vi "Set Extension.vi"(8 "error in (no error)":errorcluster, 11 "Report in":refnum<class "Wind Report.lvclass">) -> (0 "error out":errorcluster, 3 "Report out":refnum<class "Wind Report.lvclass">)   [LabVIEW 2009, in "Wind Report.lvclass"]
doc: "The protected method in the Wind Report class sets the file extension type in the object data for child classes.\n\nAAL 9/09"
uses:
  Wind Report.lvclass
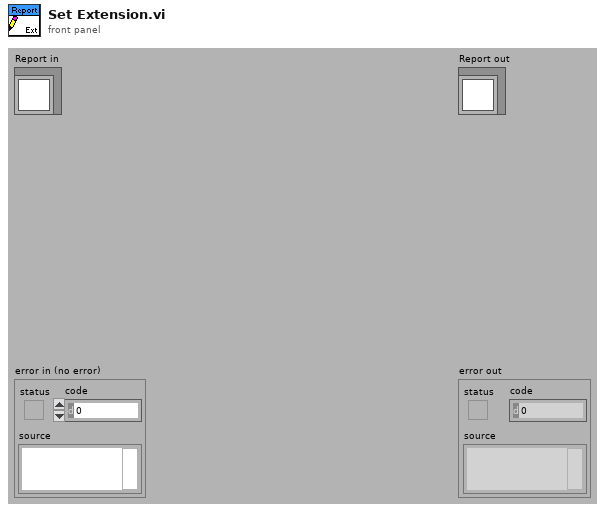
[diagram p1: front panel]
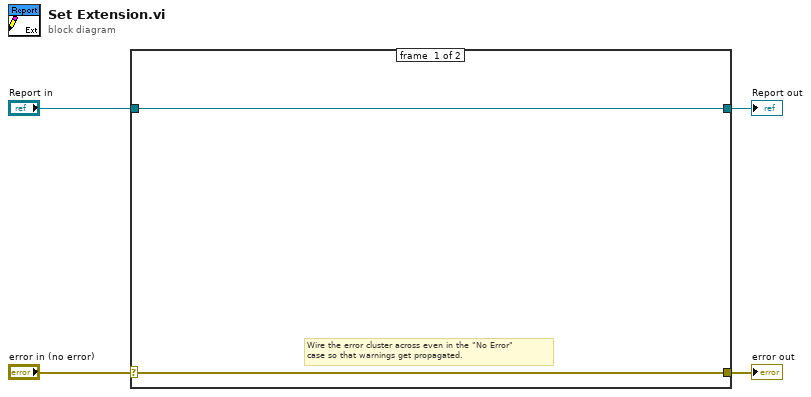
[diagram p0: block diagram]
diagram:
  n1 = case shown="No Error" "error in (no error)" {
    selector: "error in (no error)" -> [w5 w8]
    tunnel: [w5 w8] -> w3
    tunnel: [w6 w7] -> w1
    tunnel: "Report in" -> [w6 w7]
    frame #0 {
      # "Wire the error cluster across even in the \"No Error\"\ncase so that warnings get propagated."
    }
    frame #1 {
    }
  }
  "error out" <- w3
  "Report out" <- w1
